vi "Init_Data.vi"(6 "Version (no version)":string, 7 "API Root":string, 8 "error in (no error)":errorcluster, 9 "Port (protocol specific)":u16, 10 "Base URL":string, 11 "ByteGSAPIBase in":refnum<class "RESTBase.lvclass">) -> (0 "error out":errorcluster, 3 "ByteGSAPIBase out":refnum<class "RESTBase.lvclass">)   [LabVIEW 2019, in "ByteREST.lvlib" / "RESTBase.lvclass"]
doc: "Apre una nuova connessione HTTP e setta il content type a \"application/json\""
uses:
  RESTBase.lvclass
  RESTBase.lvclass/RESTBase.ctl
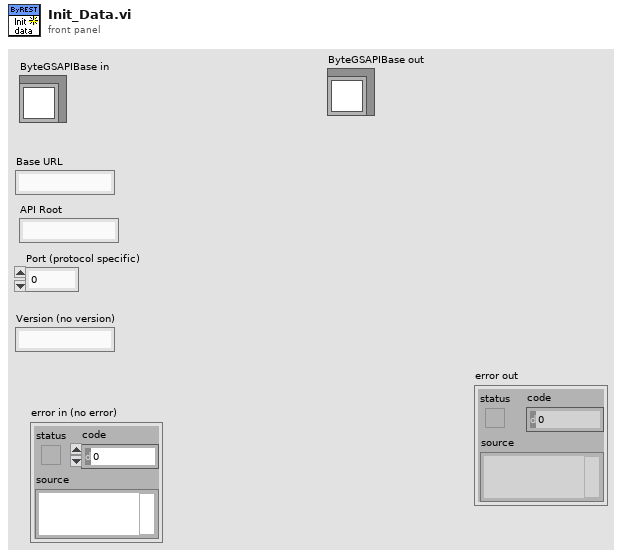
[diagram p1: front panel]
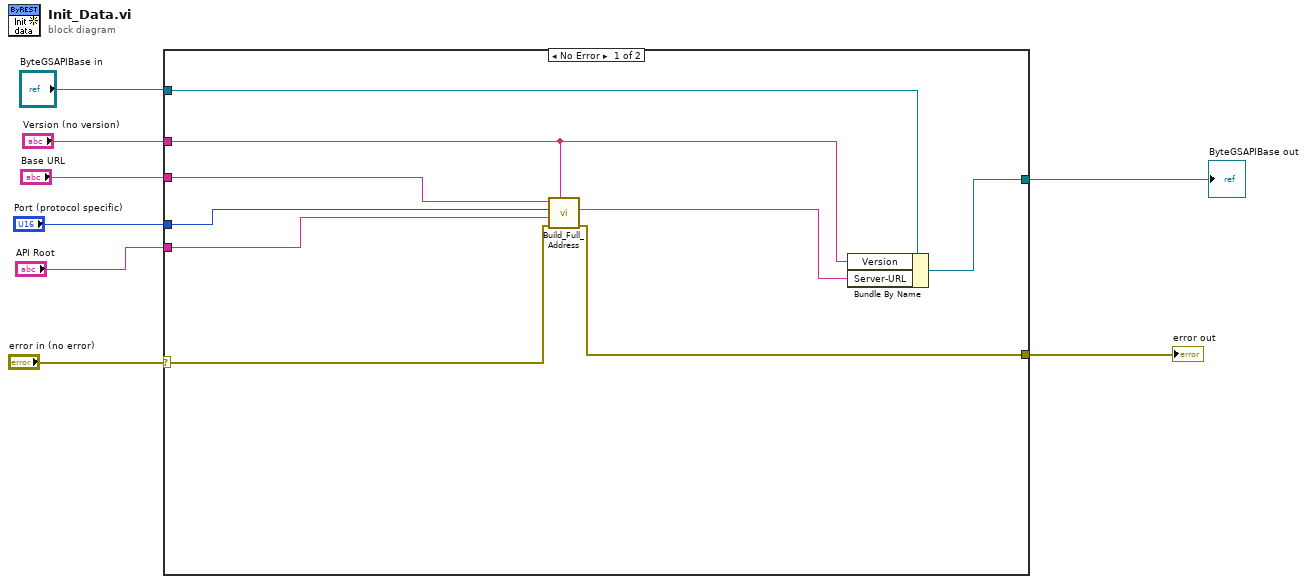
[diagram p0: block diagram]
diagram:
  n1 = case shown="No Error" "error in (no error)" {
    selector: "error in (no error)" -> [w9 w19]
    tunnel: [w10 w19] -> w7
    tunnel: [w16 w18] -> w4
    tunnel: "ByteGSAPIBase in" -> [w17 w18]
    tunnel: "Base URL" -> [w15 _]
    tunnel: "Port (protocol specific)" -> [w14 _]
    tunnel: "Version (no version)" -> [w11 _]
    tunnel: "API Root" -> [w12 _]
    frame No Error {
      n2 = call "Build_Full_Address.vi"("Version (no version)"=w11, "error in (no error)"=w9, "API Root"=w12, "Port (protocol specific)"=w14, "Base URL"=w15) -> ("error out"=w10:errorcluster, "Full URL"=w13:string)  [unwired: 5 in]
      n3 = Bundle By Name(cluster=w17, "Version"=w11, "Server-URL"=w13) -> (w16:refnum<class "RESTBase.lvclass">)
    }
    frame Error {
    }
  }
  "error out" <- w7
  "ByteGSAPIBase out" <- w4
